vi "Read Behavior.vi"(8 "error in (no error)":errorcluster, 11 "Attribute.StartupBehavior in":refnum<class "Attribute.Debug.lvclass">) -> (0 "error out":errorcluster, 2 "Behavior":T1, 3 "Attribute.StartupBehavior out":refnum<class "Attribute.Debug.lvclass">)   [LabVIEW 2019, in "SMO Debug.lvlib" / "Attribute.Debug.lvclass"]
uses:
  Attribute.Debug.lvclass
  DebugBehavior.ctl
  Attribute.Debug.lvclass/Attribute.Debug.ctl
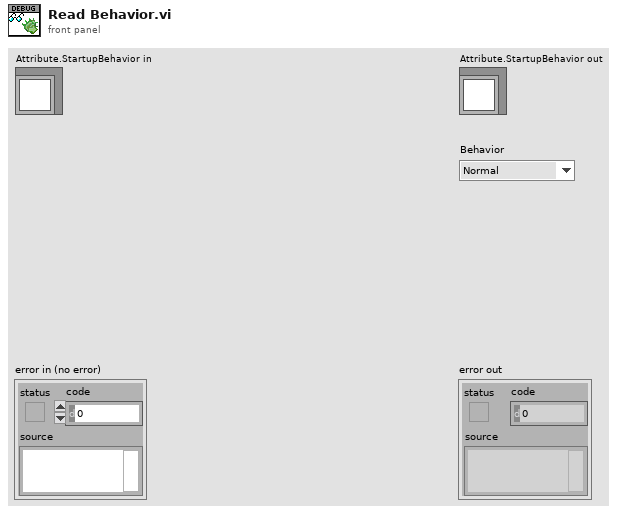
[diagram p1: front panel]
types:
  T1 = typedef "SMO Debug.lvlib/Attribute.Debug.lvclass/DebugBehavior.ctl" = enum16{"Normal", "Debug"}
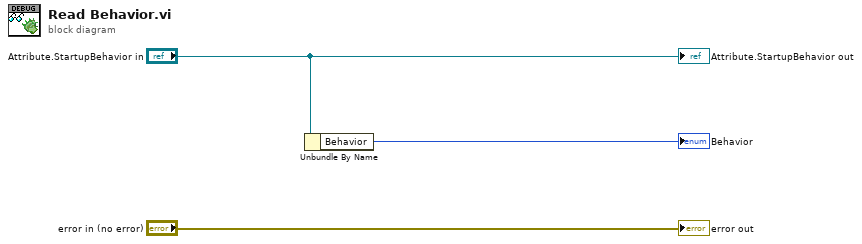
[diagram p0: block diagram]
diagram:
  n1 = Unbundle By Name("Attribute.StartupBehavior in") -> ("Behavior"=→"Behavior":T1)
  "error out" <- "error in (no error)"
  "Attribute.StartupBehavior out" <- "Attribute.StartupBehavior in"
